vi "Record 2.vi"() -> ()   [LabVIEW 2012]
uses:
  <vilib>/userdefined/High Color/IMAQdx.ctl
  <vilib>/vision/driver/NI_Vision_Acquisition_Software.lvlib
panel:
  out "Data":dynamicdata(graph)
  out "Image":T1(plugin-control)
  in  "Duration":u32=30
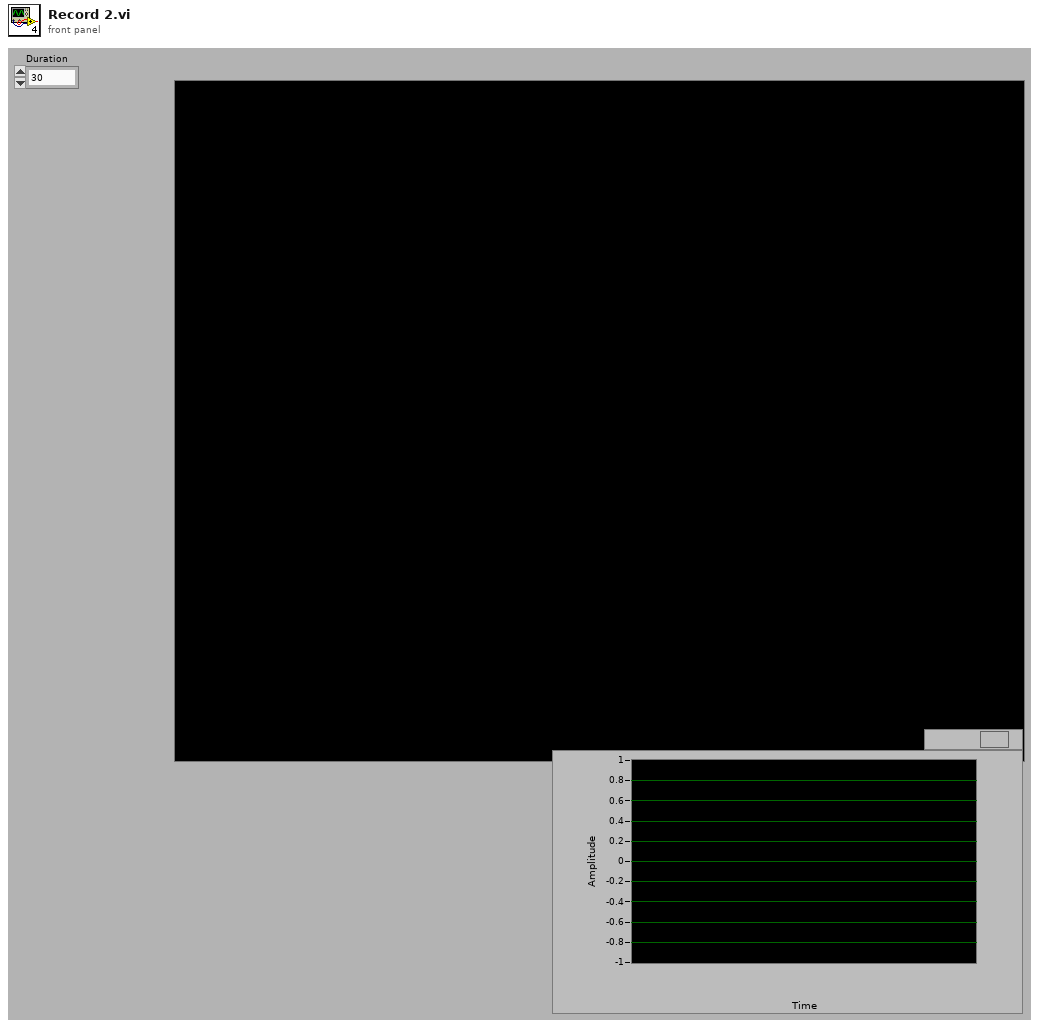
[diagram p1: front panel]
types:
  T1 = typedef "IMAQ Image.ctl" = refnum<image>
  T2 = typedef "IMAQdx.ctl" = refnum<k21>
  T3 = typedef "AviRefnum.ctl" = refnum<k1>
  T4 = typedef "Image Type" = u32
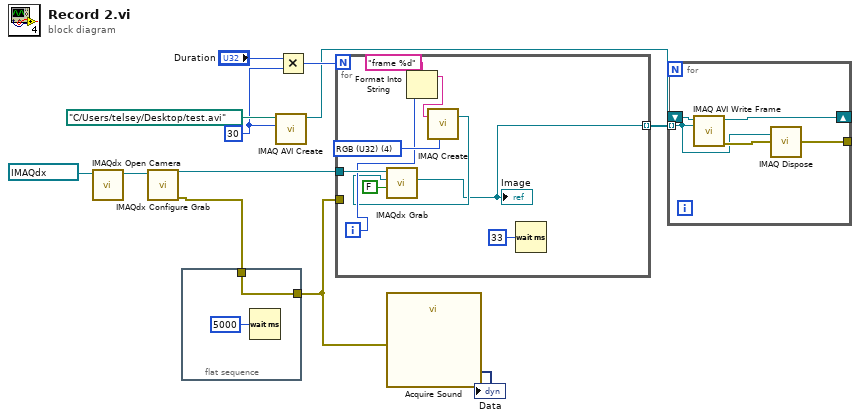
[diagram p0: block diagram]
diagram:
  w10 = u32 30 ("Frames Per Second")
  n1 = call <vilib>:"IMAQdx Open Camera.vi"("Session In"=T2 "webcam") -> ("Session Out"=w7:T2)  [unwired: 9 in, 1 out]
  n2 = call <vilib>:"IMAQdx Configure Grab.vi"("Session In"=w7) -> ("error out"=w5:errorcluster, "Session Out"=w6:T2)  [unwired: 9 in]
  n3 = flat-sequence {
    tunnel: [w13] -> w4
    tunnel: w5 -> [w13]
    frame #0 {
      n4 = Wait (ms)(milliseconds to wait=u32 5000) -> ()  [unwired: 1 out]
    }
  }
  n5 = call "IMAQ AVI Create"("Frames Per Second"=w10, "AVI Path"=path "C:/Users/telsey/Desktop/test.avi") -> ("Avi Refnum"=w2:T3)  [unwired: 8 in, 1 out]
  n6 = Multiply(x="Duration", y=w10) -> (x*y=w11:u32)
  n7 = for {
    N: w11 -> [_]
    tunnel: w6 -> [w23]
    tunnel: w4 -> [_]
    tunnel: [w15] -> w1 mode=indexing
    i -> [w18]
    w20 = T4 4 items=["Grayscale (U8)", "Grayscale (I16)", "Grayscale (SGL)", "Complex (CSG)", "RGB (U32)", "HSL (U32)", "RGB (U64)", "Grayscale (U16)"] ("Image Type")
    n8 = Format Into String(format string="frame %d", w18) -> (resulting string=w17:string)  [unwired: 2 in, 1 out]
    n9 = call "IMAQ Create"("Image Name"=w17, "Image Type"=w20) -> ("New Image"=w16:T1)  [unwired: 3 in, 1 out]
    n10 = call <vilib>:"IMAQdx Grab.vi"("Wait for Next Buffer? (Yes)"=FALSE, "Image In"=w16, "Session In"=w23) -> ("Image Out"=w15:T1)  [unwired: 5 in, 3 out]
    "Image" <- w15
    n11 = Wait (ms)(milliseconds to wait=u32 33) -> ()  [unwired: 1 out]
  }
  n12 = call "Acquire Sound"("error in (no error)"=w4) -> ("Data"=→"Data":dynamicdata)  [unwired: 17 in, 1 out]
  n13 = for {
    tunnel: w1 -> [w24] mode=indexing
    shift-right: [w26] -> _
    shift-left: w2 -> [w27]
    tunnel: [w25] -> _
    n14 = call "IMAQ AVI Write Frame"("Image"=w24, "Avi Refnum"=w27) -> ("error out"=w25:errorcluster, "Avi Refnum (duplicate)"=w26:T3)  [unwired: 8 in]
    n15 = call "IMAQ Dispose"("Image"=w24) -> ()  [unwired: 5 in, 1 out]
  }
